vi "getCommandEvents.vi"(8 "error in (no error)":errorcluster, 11 "SettingsViewer.lvclass in":refnum<class "settingsViewer.lvclass">) -> (0 "error out":errorcluster, 2 "CommandEvents.lvclass":refnum<class "CommandEvents.lvclass">, 3 "SettingsViewer.lvclass out":refnum<class "settingsViewer.lvclass">)   [LabVIEW 2009, in "Views.lvlib" / "SettingsViewer.lvclass"]
uses:
  settingsViewer.lvclass
  CommandProcessor/CommandEvents/CommandEvents.lvclass
  settingsViewer.lvclass/settingsViewer.ctl
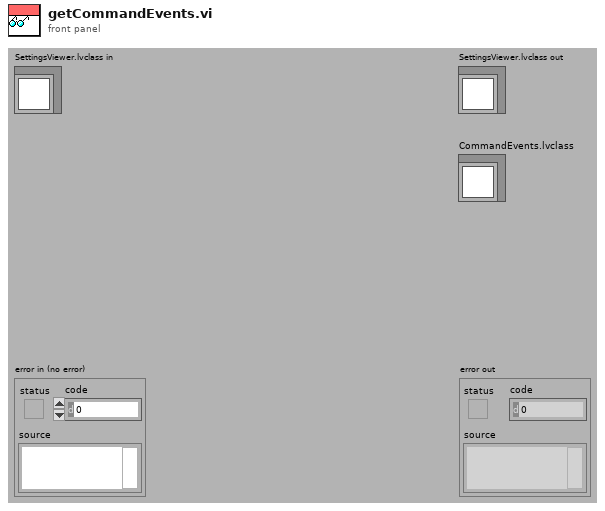
[diagram p1: front panel]
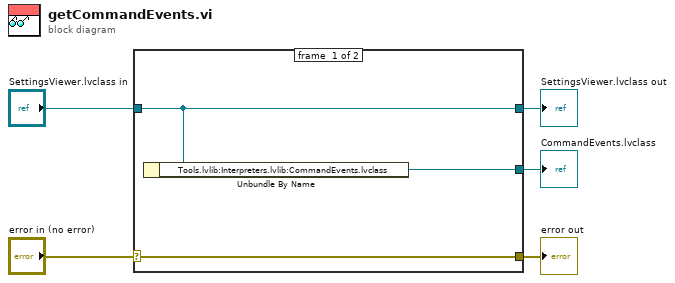
[diagram p0: block diagram]
diagram:
  n1 = case shown="No Error" "error in (no error)" {
    selector: "error in (no error)" -> [w8 w9]
    tunnel: [w8 w9] -> w4
    tunnel: [w7 w10] -> w2
    tunnel: "SettingsViewer.lvclass in" -> [w7 w10]
    tunnel: [w6 _] -> w1
    frame #0 {
      n2 = Unbundle By Name(w7) -> ("Tools.lvlib:Interpreters.lvlib:CommandEvents.lvclass"=w6:refnum<class "CommandEvents.lvclass">)
    }
    frame #1 {
    }
  }
  "error out" <- w4
  "SettingsViewer.lvclass out" <- w2
  "CommandEvents.lvclass" <- w1
